vi "Sine_wave Init 1d LUT.vi"() -> (3 "Init Data Out":u16[](array[numeric]))   [LabVIEW 2018]
uses:
  <vilib>/measure/NI_MABase.lvlib
panel:
  out "Waveform Graph - Dark":u16[](graph)
  out "size(s)":i32
  in  "DC offset":dbl
  in  "Meas Time (sec)":dbl
  in  "dt FPGA (sec)":dbl
  in  "amplitude\n[V]":dbl
  in  "Frequency \n[1/s]":dbl
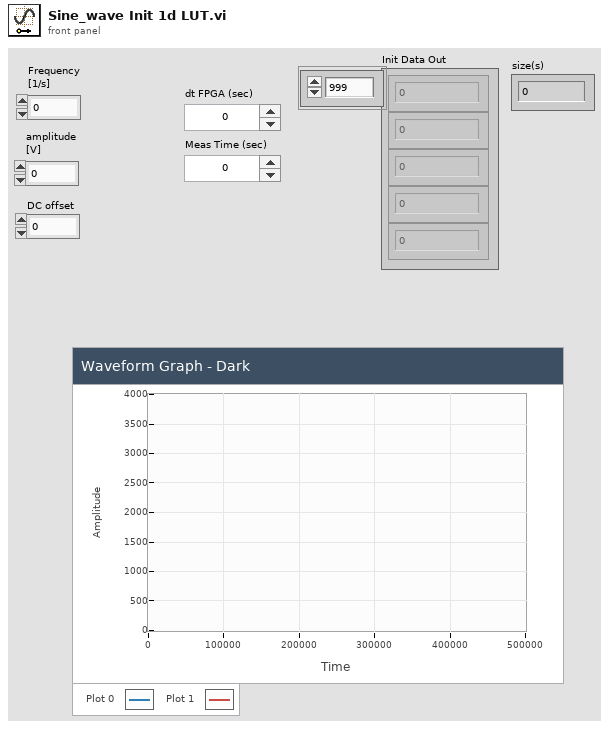
[diagram p1: front panel]
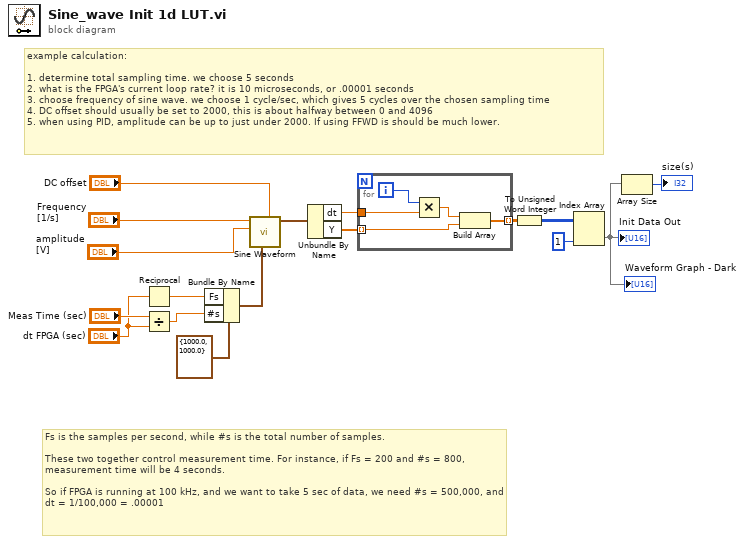
[diagram p0: block diagram]
diagram:
  # "example calculation:\n\n1. determine total sampling time. we choose 5 seconds\n2. what is the FPGA's current loop rate? it is 10 microseconds, or .00001 seconds\n3. choose frequency of sine wave. we choose 1 cycle/sec, which gives 5 cycles over the chosen sampling time\n4. DC offset should usually be set to 2000, this is about halfway between 0 and 4096\n5. when using PID, amplitude can be up to just under 2000. If using FFWD is should be much lower."
  # "Fs is the samples per second, while #s is the total number of samples.\n\nThese two together control measurement time. For instance, if Fs = 200 and #s = 800, measurement time will be 4 seconds.\n\nSo if FPGA is running at 100 kHz, and we want to take 5 sec of data, we need #s = 500,000, and dt = 1/100,000 = .00001"
  n1 = Reciprocal(x="dt FPGA (sec)") -> (1/x=w3:dbl)
  n2 = Divide(x="Meas Time (sec)", y="dt FPGA (sec)") -> (x/y=w11:dbl)
  n3 = Bundle By Name(cluster=cluster{"Fs":dbl, "#s":dbl} {"Fs"=1000.0, "#s"=1000.0} ("sampling info"), "Fs"=w3, "#s"=w11) -> (w10:cluster{"Fs":dbl, "#s":dbl})
  n4 = call <vilib>:"Sine Waveform.vi"("offset"="DC offset", "sampling info"=w10, "amplitude"="amplitude\n[V]", "frequency"="Frequency \n[1/s]") -> ("signal out"=w17:waveform(dbl))  [unwired: 6 in, 1 out]
  n5 = Unbundle By Name(w17) -> ("dt"=w14:dbl, "Y"=w5:dbl[])
  n6 = for {
    tunnel: w5 -> [w22] mode=indexing
    tunnel: w14 -> [w20]
    tunnel: [w18] -> w8 mode=indexing
    i -> [w21]
    n7 = Multiply(x=w21, y=w20) -> (x*y=w19:dbl)
    n8 = Build Array(w19, w22) -> (w18:dbl[])
  }
  n9 = To Unsigned Word Integer(number=w8) -> (unsigned 16bit integer=w7:u16[][])
  n10 = Index Array(array=w7, index (col)=1 ("disabled index (col)")) -> (element=w1:u16[])  [unwired: 1 in]
  "Init Data Out" <- w1
  "Waveform Graph - Dark" <- w1
  n11 = Array Size(array=w1) -> (size(s)=→"size(s)":i32)
